vi "DefaultSavingPath.vi"() -> ()   [LabVIEW 2018, in "RW_Protocols.lvlib"]
uses:
  RW_Protocols.lvlib
panel:
  in  "default path":string="D:\\Data\\Mai\\"
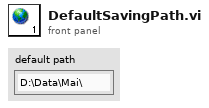
[diagram p1: front panel]
diagram:
